vi "Log Data.vi"(7 "Command":T1, 8 "error in (no error)":errorcluster, 9 "Zone":i32, 10 "Status":string, 11 "file path":path) -> (0 "error out":errorcluster)   [LabVIEW 2013]
doc: "This subVI is use to log the data to the Security log.txt file\nIt is -\n-Initializing the file path\n-Write the data\n-Stop the file path."
uses:
  Log File States.ctl
  <vilib>/Utility/file.llb/Write To Spreadsheet File (string).vi
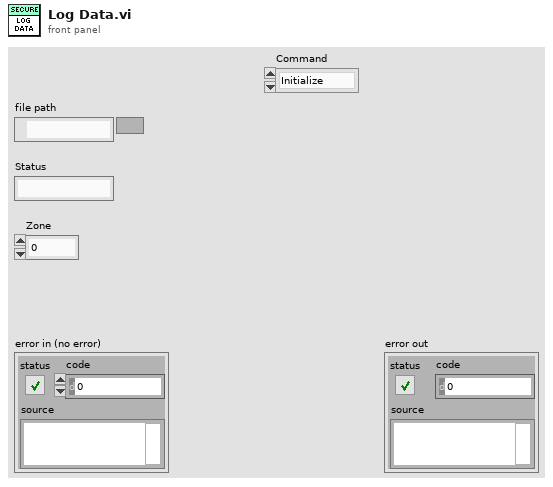
[diagram p1: front panel]
types:
  T1 = typedef "Log File States.ctl" = enum16{"Initialize", "Write", "Stop"}
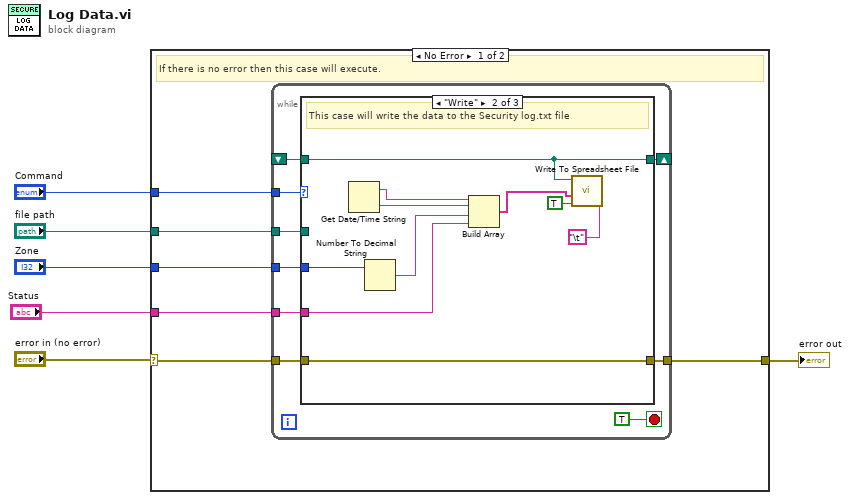
[diagram p0: block diagram]
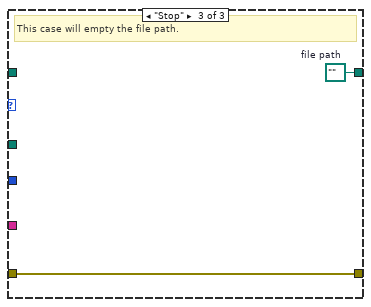
[diagram p3: hidden frame]
diagram:
  n1 = case shown="No Error" "error in (no error)" {
    selector: "error in (no error)" -> [w9 w36]
    tunnel: "Command" -> [w12 _]
    tunnel: "file path" -> [w7 _]
    tunnel: "Status" -> [w11 _]
    tunnel: "Zone" -> [w10 _]
    tunnel: [w8 w36] -> w6
    frame No Error {
      # "If there is no error then this case will execute."
      n2 = while {
        tunnel: w12 -> [w20]
        tunnel: w7 -> [w19]
        shift-right: [w18] -> _
        shift-left: _ -> [w17]
        tunnel: w11 -> [w16]
        tunnel: w10 -> [w15]
        tunnel: w9 -> [w14]
        tunnel: [w13] -> w8
        stop <- TRUE stop-if-true
        n3 = case shown="\"Write\"" w20 {
          tunnel: w19 -> [w23 _ _]
          tunnel: [w23 w33 w35] -> w18
          tunnel: w17 -> [_ w33 _]
          tunnel: w16 -> [_ w24 _]
          tunnel: w15 -> [_ w30 _]
          tunnel: w14 -> [w22 w29 w34]
          tunnel: [w22 w29 w34] -> w13
          frame "Initialize", Default {
            # "Stoaring the file path to the shift register."
            # "This case will initialize the file path."
          }
          frame "Write" {
            # "This case will write the data to the Security log.txt file"
            n4 = Get Date/Time String() -> (date string=w32:string, time string=w31:string)  [unwired: 3 in]
            n5 = Number To Decimal String(number=w30) -> (decimal integer string=w25:string)  [unwired: 1 in]
            n6 = Build Array(w32, w31, w25, w24) -> (w26:string[])
            n7 = call-poly <vilib>:"Write To Spreadsheet File.vi"("delimiter (\\t)"="\t", "append to file? (new file:F)"=TRUE, "1D data"=w26, "file path (dialog if empty)"=w33) -> ()  [unwired: 4 in, 1 out]
          }
          frame "Stop" {
            w35 = path ""  # file path
            # "This case will empty the file path."
          }
        }
      }
    }
    frame Error {
      # "If there is error then this case will execute."
    }
  }
  "error out" <- w6
